vi "Script Find current Error Codes.vi"(8 "error in":errorcluster, 11 "Library in":refnum<vi>) -> (0 "error out":errorcluster, 2 "Error Codes and Descriptions":T1[](array[typedef]), 3 "Library out":refnum<vi>)   [LabVIEW 2019, in "Panther Dashboard.lvlib"]
uses:
  Panther Dashboard.lvlib
  Error Code and Description--cluster.ctl
  <vilib>/Utility/traverseref.llb/TRef TravTarget.ctl
  <vilib>/Utility/traverseref.llb/VI Scripting - Traverse.lvlib
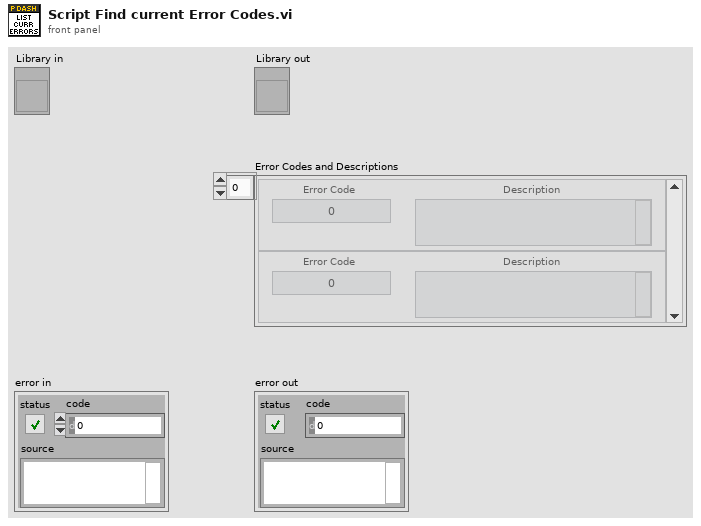
[diagram p1: front panel]
types:
  T1 = typedef "Panther Dashboard.lvlib/Error Code and Description--cluster.ctl" = cluster{"Error Code":i32, "Description":string}
  T2 = typedef "TRef TravTarget.ctl" = enum16{"FP", "BD", "Other"}
  T3 = cluster{"Clipped Error Description":string, "Full Error Description":string, "code":i32, "Family":string, "Custom Description":string, "Is Error":bool, "Types":variant[], "Include Call Chain?":bool, "Error Text Visible":bool}
  T4 = cluster{"Library Version":cluster{"Major":u16, "Minor":u16, "Fix":u16, "Build":u16}, "State":variant}
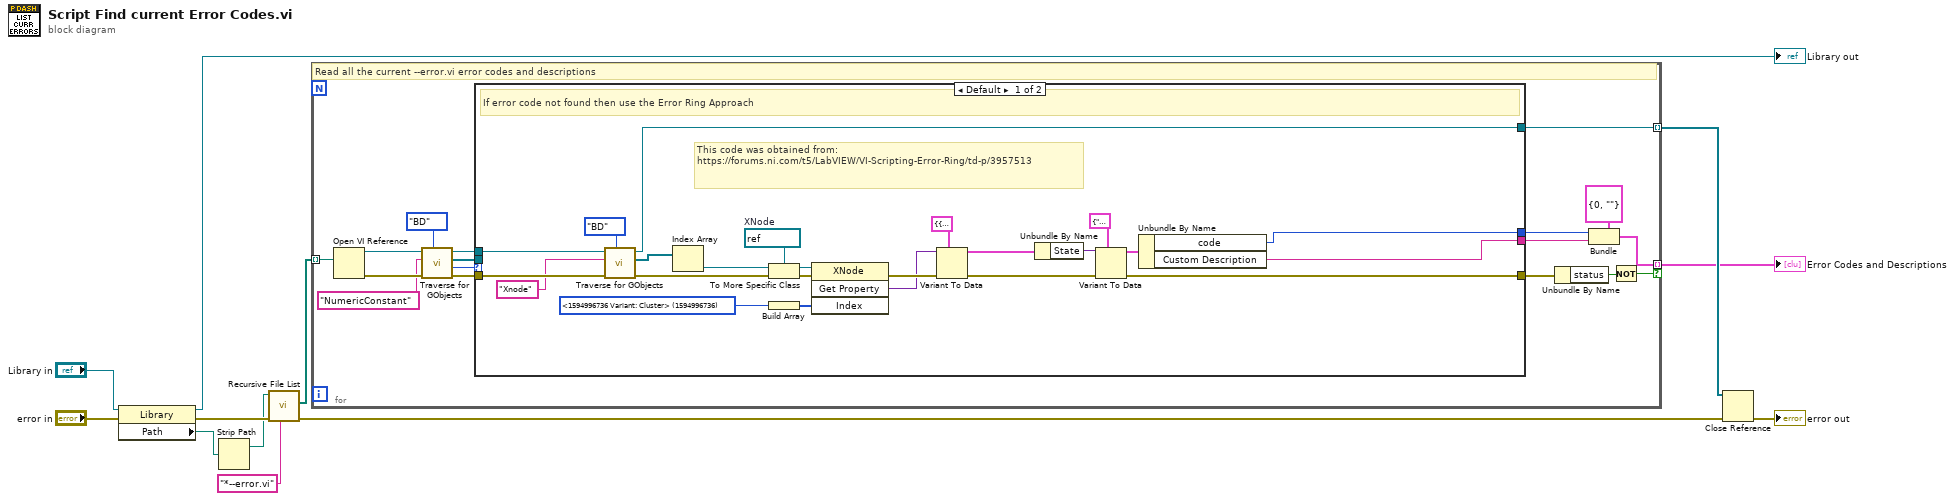
[diagram p0: block diagram]
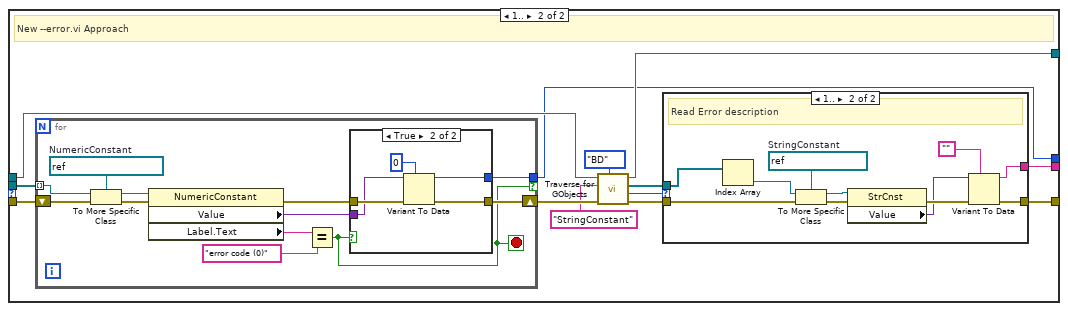
[diagram p2: hidden frame]
diagram:
  n1 = property class="Library"(reference="Library in", error in="error in") -> (reference out=→"Library out":refnum<vi>, error out=w11:errorcluster, "Path"=w2:path)
  n2 = Strip Path(path=w2) -> (stripped path=w7:path)  [unwired: 1 out]
  n3 = call <vilib>:"Recursive File List.vi"("pattern"="*--error.vi", "error in (no error)"=w11, "Folder Path"=w7) -> ("error out"=w10:errorcluster, "All Files in Dir"=w5:path[])  [unwired: 4 in, 3 out]
  n4 = for {
    tunnel: w5 -> [w17] mode=indexing
    tunnel: [w15] -> w4 mode=indexing
    tunnel: [w16] -> w3 mode=indexing if=w14
    # "Read all the current --error.vi error codes and descriptions"
    n5 = Open VI Reference(vi path=w17) -> (vi reference=w24:refnum<vi>, error out=w28:errorcluster)  [unwired: 5 in]
    n6 = call <vilib>:"Traverse for GObjects.vi"("Traverse Target"=TRef_TravTarget."BD", "error in (no error)"=w28, "Class Name"="NumericConstant", "VI Refnum"=w24) -> ("error out"=w29:errorcluster, "# of Refs"=w20:i32, "References"=w25:refnum<vi>[], "dup VI Refnum"=w19:refnum<vi>)  [unwired: 4 in]
    n7 = case shown="Default" w20 {
      tunnel: [w32 w54] -> w23
      tunnel: [w50 w65] -> w27
      tunnel: w29 -> [w53 w64]
      tunnel: w25 -> [_ w62]
      tunnel: w19 -> [w45 w57]
      tunnel: [w31 w56] -> w18
      tunnel: [w30 w55] -> w15
      frame Default {
        w41 = u32 1594996736 items=["<1594996736 Variant: Cluster>"=1594996736, "<1594996767 Diagram RefNum>"=1594996737, "<1594996738 ProjectItem Refnum>"=1594996738, "<1594996739 Boolean>"=1594996739, "<1594996740 Boolean>"=1594996740, "<1594996741 Boolean>"=1594996741, "<1594996742 String: .html file name>"=1594996742, "<1594996743 Help Path>"=1594996743, "<1594996744 String: Tip Strip>"=1594996744, "<1594996745 Boolean>"=1594996745, "<104204298 Boolean>"=104204298, "AutoSize To Fit Contents?"=104204288, "Basic Object Flags"=103983116, "Bounds"=103983107, "Bounds:Area Height"=103983109, "Bounds:Area Width"=103983108, "Breakpoint Status"=104173580, "Clump Num"=104173572, "Content Rect"=104204293, "Description"=104173570, "Diagrams[]"=104204291, "Fire Count"=104173574, "Fix Contents"=104204297, "Frame Size"=104204290, "Icon"=104173576, "Is Asynchronous"=104173575, "Is Break Point Set"=104173571, "Is Run At Any Loop"=104173578, "Is Wizard Locked"=103983117, "Label"=104173569, "Master Bounds Rect"=103983115, "Position"=103983104, "Position:Left"=103983105, "Position:Top"=103983106, "Resize Info:Can Resize Horizontally"=103983119, "Resize Info:Can Resize Vertically"=103983120, "Resize Info:Include In Resize"=103983122, "Resize Info:Name in Resize Dialog"=103983121, "Selected"=103983113, "Shared Clones:Automatic Allocation Strategy Enabled"=104204295, "Shared Clones:Pre-Allocate"=104204296, "Short Count"=104173573, "Style"=104173577, "Target Syntax Checking"=104204292, "Terminals[]"=104173568, "Total Bounds Rect"=103983114, "Tunnels[]"=104204289, "UID"=103983123]
        w44 = refnum<vi> refnum  # XNode
        # "This code was obtained from:\nhttps://forums.ni.com/t5/LabVIEW/VI-Scripting-Error-Ring/td-p/3957513"
        # "If error code not found then use the Error Ring Approach"
        n8 = call <vilib>:"Traverse for GObjects.vi"("Traverse Target"=TRef_TravTarget."BD", "error in (no error)"=w53, "Class Name"="Xnode", "VI Refnum"=w45) -> ("error out"=w52:errorcluster, "References"=w43:refnum<vi>[], "dup VI Refnum"=w30:refnum<vi>)  [unwired: 4 in, 1 out]
        n9 = Index Array(array=w43) -> (element=w42:refnum<vi>)  [unwired: 1 in]
        n10 = To More Specific Class(target class=w44, reference=w42, error in=w52) -> (specific class reference=w40:refnum<vi>, error out=w51:errorcluster)
        n11 = Build Array(w41) -> (w39:u32[])
        n12 = invoke class="XNode" method="Get Property"(reference=w40, error in=w51, "Index"=w39) -> (error out=w49:errorcluster, "GetProperty"=w34:variant)  [unwired: 1 in, 2 out]
        n13 = Variant To Data(error in=w49, type=T4 {"Library Version"={"Major"=0, "Minor"=0, "Fix"=0, "Build"=0}, "State"=variant} ("output cluster"), Variant=w34) -> (data=w38:T4, error out=w48:errorcluster)
        n14 = Unbundle By Name(w38) -> ("State"=w36:variant)
        n15 = Variant To Data(error in=w48, type=T3 {"Clipped Error Description"="", "Full Error Description"="", "code"=0, "Family"="", "Custom Description"="", "Is Error"=TRUE, "Types"=[], "Include Call Chain?"=TRUE, "Error Text Visible"=TRUE} ("State"), Variant=w36) -> (data=w33:T3, error out=w50:errorcluster)
        n16 = Unbundle By Name(w33) -> ("code"=w32:i32, "Custom Description"=w31:string)
      }
      frame 1.. {
        # "New --error.vi Approach"
        n17 = for {
          tunnel: w62 -> [w74] mode=indexing
          tunnel: [w68] -> w54 if=w67
          shift-right: [w75] -> w63
          shift-left: w64 -> [w78]
          stop <- w67 stop-if-true
          w73 = refnum<vi> refnum  # NumericConstant
          n18 = To More Specific Class(target class=w73, reference=w74, error in=w78) -> (specific class reference=w72:refnum<vi>, error out=w77:errorcluster)
          n19 = property class="NumericConstant"(reference=w72, error in=w77) -> (error out=w76:errorcluster, "Value"=w69:variant, "Label.Text"=w71:string)  [unwired: 1 out]
          n20 = Equal?(x=w71, y="error code (0)") -> (x = y?=w67:bool)
          n21 = case shown="True" w67 {
            tunnel: w69 -> [_ w81]
            tunnel: w76 -> [w79 w84]
            tunnel: [w79 w83] -> w75
            tunnel: [_ w80] -> w68
            frame False {
            }
            frame True {
              n22 = Variant To Data(error in=w84, type=0, Variant=w81) -> (data=w80:i32, error out=w83:errorcluster)
            }
          }
        }
        n23 = call <vilib>:"Traverse for GObjects.vi"("Traverse Target"=TRef_TravTarget."BD", "error in (no error)"=w63, "Class Name"="StringConstant", "VI Refnum"=w57) -> ("error out"=w66:errorcluster, "# of Refs"=w58:i32, "References"=w61:refnum<vi>[], "dup VI Refnum"=w55:refnum<vi>)  [unwired: 4 in]
        n24 = case shown="1.." w58 {
          tunnel: [_ w92] -> w56
          tunnel: [w85 w96] -> w65
          tunnel: w66 -> [w85 w95]
          tunnel: w61 -> [_ w87]
          frame Default {
          }
          frame 1.. {
            w91 = refnum<vi> refnum  # StringConstant
            # "Read Error description"
            n25 = Index Array(array=w87) -> (element=w86:refnum<vi>)  [unwired: 1 in]
            n26 = To More Specific Class(target class=w91, reference=w86, error in=w95) -> (specific class reference=w90:refnum<vi>, error out=w94:errorcluster)
            n27 = property class="StrCnst"(reference=w90, error in=w94) -> (error out=w93:errorcluster, "Value"=w89:variant)  [unwired: 1 out]
            n28 = Variant To Data(error in=w93, type="", Variant=w89) -> (data=w92:string, error out=w96:errorcluster)
          }
        }
      }
    }
    n29 = Unbundle By Name(w27) -> ("status"=w13:bool)
    n30 = Bundle(cluster=T1 {"Error Code"=0, "Description"=""} ("Panther Dashboard.lvlib:Error Code and Description--cluster"), "Error Code"=w23, "Description"=w18) -> (w16:T1)
    n31 = Not(x=w13) -> (.not. x?=w14:bool)
  }
  "Error Codes and Descriptions" <- w3
  n32 = Close Reference(reference=w4, error in (no error)=w10) -> (error out=→"error out":errorcluster)
